vi "GateOpen.vi"   [LabVIEW 2014, in "GateLib.lvlib"]
uses:
  GateLib.lvlib
  GateRefs.ctl
  <vilib>/Rock Robotics/WPI/Solenoid/WPI_SolenoidChannel.ctl
  <vilib>/Rock Robotics/WPI/Solenoid/WPI_SolenoidOpenDouble.vi
types:
  T1 = typedef "WPI_SolenoidChannel.ctl" = enum8{"Solenoid 0", "Solenoid 1", "Solenoid 2", "Solenoid 3", "Solenoid 4", "Solenoid 5", "Solenoid 6", "Solenoid 7", "Invalid"}
  T2 = typedef "GateLib.lvlib/GateRefs.ctl" = enum16{"GateCyl"}
  T3 = typedef "WPI_SolenoidDevRef.ctl" = cluster{"DevStatus":errorcluster, "Pneumatics Control Module":u8, "Forward Solenoid Channel":T1, "Reverse Solenoid Channel":T1}
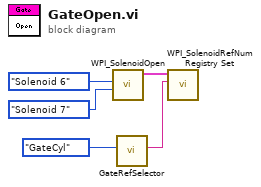
[diagram p0: block diagram]
diagram:
  n1 = call-poly <vilib>:"WPI_SolenoidOpen.vi"("Reverse Solenoid Channel"=WPI_SolenoidChannel."Solenoid 7", "Forward Solenoid Channel"=WPI_SolenoidChannel."Solenoid 6") -> ("SolenoidDevRef"=w1:T3)  [unwired: 8 in, 1 out]
  n2 = call "GateRefSelector.vi"("GateRefs"=GateRefs."GateCyl") -> ("Refnum"=w2:string)  [unwired: 10 in]
  n3 = call <vilib>:"WPI_SolenoidRefNum Registry Set.vi"("refnum name"=w2, "SolenoidDevRef"=w1) -> ()  [unwired: 8 in, 2 out]
